vi "Format Precision Query.vi"(8 "error in":errorcluster, 11 "Instrument Handle In":i32) -> (0 "error out":errorcluster, 1 "Exponent":i32, 2 "Mantissa":i32, 3 "Instrument Handle Out":i32)   [LabVIEW 8.6, in "ZTScopeM.lvlib"]
doc: "Query the data precision for all floating point values from the instrument. The precision is specified in the following format: \n\nprecision = mantissa^exponent"
uses:
  ZTScopeM.lvlib
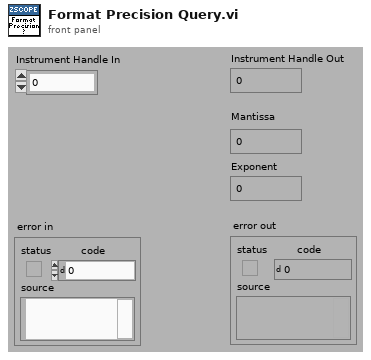
[diagram p1: front panel]
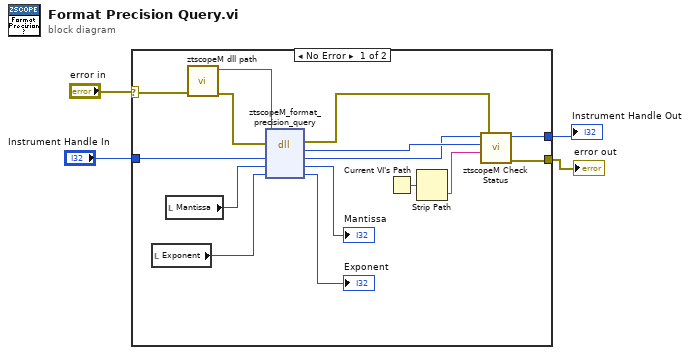
[diagram p0: block diagram]
diagram:
  n1 = case shown="No Error" "error in" {
    selector: "error in" -> [w8 w21]
    tunnel: [w10 w21] -> w1
    tunnel: "Instrument Handle In" -> [w19 w20]
    tunnel: [w9 w20] -> w3
    frame #0 {
      n2 = local read "Exponent"() -> (w16:i32)
      n3 = local read "Mantissa"() -> (w18:i32)
      n4 = call "ztscopeM dll path.vi"("error in (no error)"=w8) -> ("error out"=w6:errorcluster, "<instrument>.dll path"=w7:path)  [unwired: 9 in]
      n5 = dll-call lib="C:/Program Files (x86)/National Instruments/LabVIEW 2013/instr.lib/ztscopem/ztscopeM.dll" fn="ztscopeM_format_precision_query"(path in=w7, error in=w6, "instrument handle"=w19, "mantissa"=w18, "exponent"=w16) -> (error out=w5:errorcluster, "status"=w12:i32, "instrument handle"=w11:i32, "mantissa"=→"Mantissa":u16, "exponent"=→"Exponent":u16)  [unwired: 1 in, 1 out]
      n6 = Current VI's Path() -> (path=w14:path)
      n7 = Strip Path(path=w14) -> (name=w13:string)  [unwired: 1 out]
      n8 = call "ztscopeM Check Status.vi"("error in"=w5, "name of VI"=w13, "status (return code)"=w12, "instrument handle in"=w11) -> ("error out"=w10:errorcluster, "instrument handle out"=w9:i32)  [unwired: 2 in]
    }
    frame #1 {
    }
  }
  "Instrument Handle Out" <- w3
  "error out" <- w1
